vi "Get Scanner.vi"(8 "error in (no error)":errorcluster, 11 "Spectrometer iHR320 in":refnum<class "Spectrometer iHR320.lvclass">) -> (0 "error out":errorcluster, 2 "Default Scanner out":refnum<class "Scanner.lvclass">)   [LabVIEW 2009, in "Spectrometer iHR320.lvclass"]
doc: "(Dynamic) Returns the default Scanner object that scans over this Scannable. (Note that a Scannable may have multiple Scanners associated with it.) A Scanner is an analogue to an Iterator class in other languages."
uses:
  Spectrometer iHR320.lvclass
  Scanners/Scanner/Scanner.lvclass
  Utility Classes/Scannable/Scannable.lvclass
  Scanners/Wavelength iHR320/Wavelength iHR320.lvclass
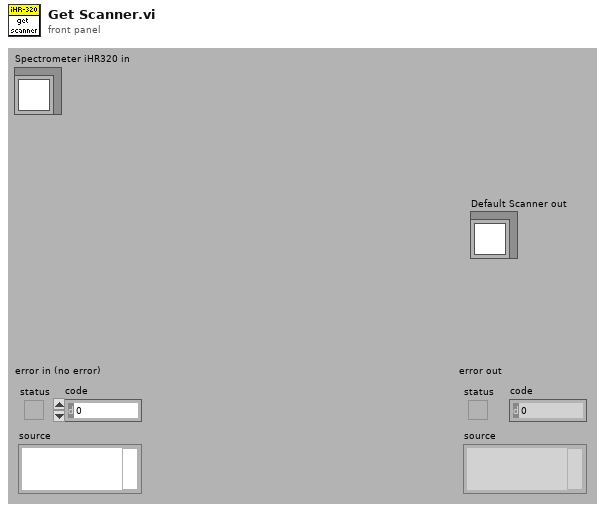
[diagram p1: front panel]
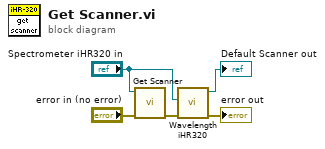
[diagram p0: block diagram]
diagram:
  n1 = call-parent "Get Scanner.vi"("error in (no error)"="error in (no error)", "Scannable in"="Spectrometer iHR320 in") -> ("error out"=w4:errorcluster)  [unwired: 8 in, 1 out]
  n2 = call "Wavelength iHR320.vi"("error in (no error)"=w4, "Spectrometer iHR320.lvclass"="Spectrometer iHR320 in") -> ("error out"=→"error out":errorcluster, "Wavelength iHR320.lvclass Out"=→"Default Scanner out":refnum<class "Wavelength iHR320.lvclass">)  [unwired: 8 in]
